vi "GT_ArcXYR.vi"(0 "rtn_In":cluster{"rtn":i16, "Func":string}, 1 "X":i32, 2 "Y":i32, 3 "radius":dbl, 5 "crd":i16, 7 "fifo":i16, 9 "VelEnd":dbl, 12 "synVel":dbl, 13 "synAcc":dbl, 14 "circleDir":i16) -> (4 "rtn_Out":cluster{"rtn":i16, "Func":string}, 6 "crd out":i16, 8 "fifo out":i16)   [LabVIEW 2014]
uses:
  VC6/gts.dll
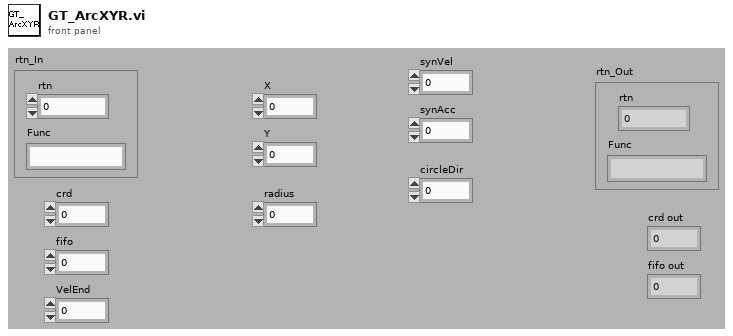
[diagram p1: front panel]
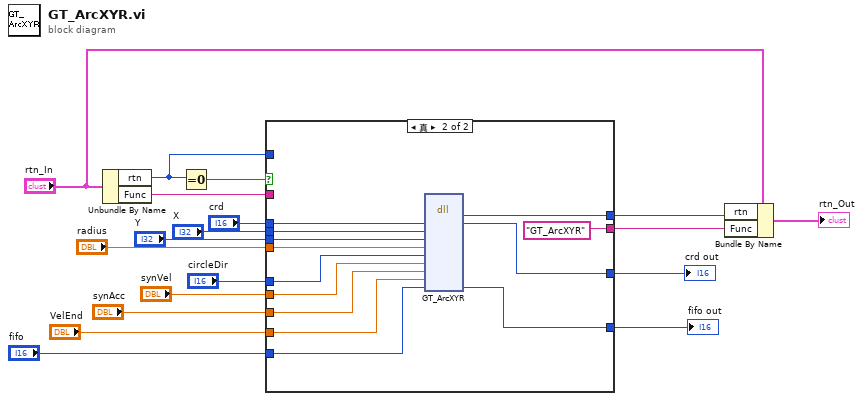
[diagram p0: block diagram]
diagram:
  n1 = Unbundle By Name("rtn_In") -> ("rtn"=w2:i16, "Func"=w1:string)
  n2 = Equal To 0?(x=w2) -> (x = 0?=w18:bool)
  n3 = case shown="真" w18 {
    tunnel: [w21 "GT_ArcXYR" ("Func")] -> w15
    tunnel: [w22 w34] -> w14
    tunnel: "crd" -> [w20 w33]
    tunnel: "X" -> [_ w32]
    tunnel: "Y" -> [_ w31]
    tunnel: "radius" -> [_ w30]
    tunnel: "circleDir" -> [_ w29]
    tunnel: "synVel" -> [_ w28]
    tunnel: "synAcc" -> [_ w27]
    tunnel: "VelEnd" -> [_ w26]
    tunnel: "fifo" -> [w19 w25]
    tunnel: [w20 w24] -> w4
    tunnel: [w19 w23] -> w3
    tunnel: w2 -> [w22 _]
    tunnel: w1 -> [w21 _]
    frame False {
    }
    frame True {
      n4 = dll-call lib="PTH2Fabs DNewGTS AC-800LWin7版源程序-20170926gts85VC6gts.dll" fn="GT_ArcXYR"("crd"=w33, "X"=w32, "Y"=w31, "radius"=w30, "circleDir"=w29, "synVel"=w28, "synAcc"=w27, "VelEnd"=w26, "fifo"=w25) -> ("rtn"=w34:i16, "crd"=w24:i16, "fifo"=w23:i16)  [unwired: 10 in, 2 out]
    }
  }
  "crd out" <- w4
  "fifo out" <- w3
  n5 = Bundle By Name(cluster="rtn_In", "rtn"=w14, "Func"=w15) -> (→"rtn_Out":cluster{"rtn":i16, "Func":string})
